vi "8.8.2_b.vi"() -> ()   [LabVIEW 2018]
panel:
  out "a":dbl(graph)
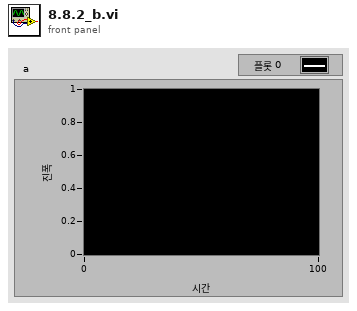
[diagram p1: front panel]
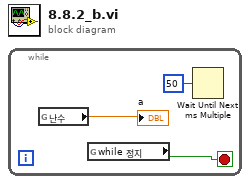
[diagram p0: block diagram]
diagram:
  n1 = while {
    stop <- w1 stop-if-true
    n2 = global read "8.8.2_글로벌.vi" "난수"() -> (→"a":dbl)
    n3 = global read "8.8.2_글로벌.vi" "while 정지"() -> (w1:bool)
    n4 = Wait Until Next ms Multiple(millisecond multiple=u32 50 ("ms 배수")) -> ()  [unwired: 1 out]
  }
